vi "Msg.vi"(7 "Actor in":refnum<class "Actor.lvclass">, 11 "Last Ack Msg in":refnum<class "Last Ack Msg.lvclass">) -> (0 "error out":errorcluster, 2 "Destroy Self?":bool, 5 "Actor out":refnum<class "Actor.lvclass">)   [LabVIEW 2021, in "Last Ack.lvlib" / "Last Ack Msg.lvclass"]
uses:
  Last Ack Msg.lvclass
  AAM/Actor/Actor.lvclass
  Last Ack/Last Ack.lvclass
  Last Ack Msg.lvclass/Last Ack Msg.ctl
  a3ac8300-150d-432b-8cde-d5f903e50042.vi
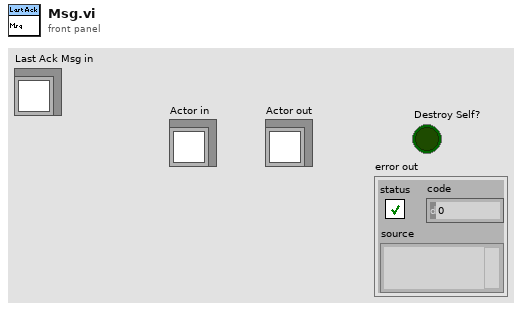
[diagram p1: front panel]
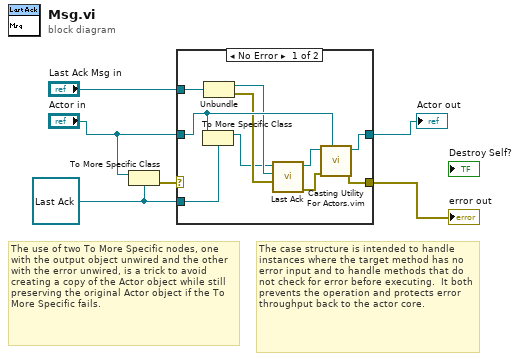
[diagram p0: block diagram]
diagram:
  w1 = refnum<class "Last Ack.lvclass"> refnum ("Last Ack.lvlib:Last Ack.lvclass")
  # "The use of two To More Specific nodes, one with the output object unwired and the other with the error unwired, is a trick to avoid creating a copy of the Actor object while still preserving the original Actor object if the To More Specific fails."
  # "The case structure is intended to handle instances where the target method has no error input and to handle methods that do not check for error before executing.  It both prevents the operation and protects error throughput back to the actor core."
  n1 = To More Specific Class(target class=w1, reference="Actor in") -> (error out=w6:errorcluster)  [unwired: 1 in, 1 out]
  n2 = case shown="No Error" w6 {
    selector: w6 -> [_ w18]
    tunnel: [w13 w18] -> w4
    tunnel: [w14 w17] -> w2
    tunnel: "Actor in" -> [w15 w17]
    tunnel: w1 -> [w16 _]
    tunnel: "Last Ack Msg in" -> [w12 _]
    frame No Error {
      n3 = To More Specific Class(target class=w16, reference=w15) -> (specific class reference=w7:refnum<class "Last Ack.lvclass">)  [unwired: 1 in, 1 out]
      n4 = Unbundle(w12) -> (w8:refnum<class "Actor.lvclass">, w9:errorcluster)
      n5 = call-dynamic "Last Ack.vi"("Error"=w9, "Actor"=w8, "Last Ack in"=w7) -> ("error out"=w10:errorcluster, "Last Ack out"=w11:refnum<class "Last Ack.lvclass">)  [unwired: 7 in]
      n6 = call "Casting Utility For Actors.vim"("type"=w15, "error in (no error)"=w10, "Actor in"=w11) -> ("error out"=w13:errorcluster, "Actor out"=w14:refnum<class "Actor.lvclass">)  [unwired: 7 in]
    }
    frame Error {
      # "If type check fails, pass the original object out again."
    }
  }
  "error out" <- w4
  "Actor out" <- w2
